vi "opCRD Server.vi"   [LabVIEW 2013]
uses:
  CRD/tCRD.lvclass
  Reusable/Instrument/state.ctl
  Reusable/Instrument/Instrument.lvclass
types:
  T1 = typedef "Instrument.lvclass/state.ctl" = enum8{"Configure", "Acquire", "Wait", "Quit", "Handle Error", "NOOP"}
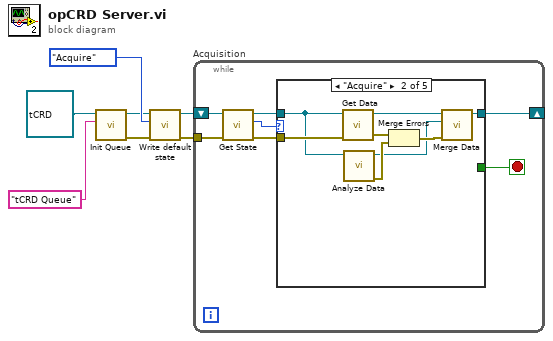
[diagram p0: block diagram]
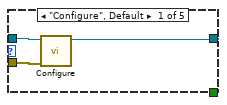
[diagram p2: hidden frame]
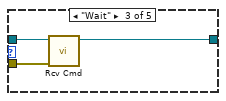
[diagram p3: hidden frame]
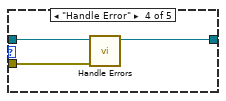
[diagram p4: hidden frame]
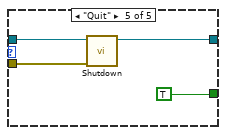
[diagram p5: hidden frame]
diagram:
  n1 = call "Init Queue.vi"("queue_name"="tCRD Queue", "Instrument in"=refnum<class "tCRD.lvclass"> refnum ("tCRD")) -> ("error out"=w1:errorcluster, "Instrument out"=w2:refnum<class "tCRD.lvclass">)  [unwired: 8 in]
  n2 = call "Write default state.vi"("error in (no error)"=w1, "instr state"=state."Acquire", "Instrument in"=w2) -> ("error out"=w3:errorcluster, "Instrument out"=w4:refnum<class "tCRD.lvclass">)  [unwired: 7 in]
  n3 = while "Acquisition" {
    tunnel: w3 -> [w14]
    shift-right: [w8] -> _
    shift-left: w4 -> [w12]
    stop <- w9 stop-if-true
    n4 = call "Get State.vi"("error in"=w14, "Instrument in"=w12) -> ("error out"=w10:errorcluster, "default state"=w13:T1, "Instrument out"=w11:refnum<class "tCRD.lvclass">)  [unwired: 7 in]
    n5 = case shown="\"Acquire\"" w13 {
      tunnel: w11 -> [w17 w18 w28 w31 w34]
      tunnel: w10 -> [w16 w25 w26 w30 w33]
      tunnel: [_ _ _ _ TRUE] -> w9
      tunnel: [w15 w21 w27 w29 w32] -> w8
      frame "Configure", Default {
        n6 = call-dynamic "Configure.vi"("error in"=w16, "tCRD in"=w17) -> ("tCRD out"=w15:refnum<class "tCRD.lvclass">)  [unwired: 8 in, 1 out]
      }
      frame "Acquire" {
        n7 = call-dynamic "Get Data.vi"("error in"=w25, "tCRD in"=w18) -> ("error out"=w24:errorcluster, "tCRD out"=w22:refnum<class "tCRD.lvclass">)  [unwired: 8 in]
        n8 = call-dynamic "Analyze Data.vi"("tCRD in"=w18) -> ("error out"=w23:errorcluster, "tCRD out"=w19:refnum<class "tCRD.lvclass">)  [unwired: 9 in]
        n9 = Merge Errors(w24, w23) -> (w20:errorcluster)
        n10 = call-dynamic "Merge Data.vi"("error in"=w20, "Analyzed"=w19, "Acquired"=w22) -> ("tCRD out"=w21:refnum<class "tCRD.lvclass">)  [unwired: 7 in, 1 out]
      }
      frame "Wait" {
        n11 = call-dynamic "Rcv Cmd.vi"("error in"=w26, "tCRD in"=w28) -> ("tCRD out"=w27:refnum<class "tCRD.lvclass">)  [unwired: 8 in, 1 out]
      }
      frame "Handle Error" {
        n12 = call-dynamic "Handle Errors.vi"("error in"=w30, "tCRD in"=w31) -> ("tCRD out"=w29:refnum<class "tCRD.lvclass">)  [unwired: 7 in, 2 out]
      }
      frame "Quit" {
        n13 = call-dynamic "Shutdown.vi"("error in"=w33, "tCRD in"=w34) -> ("tCRD out"=w32:refnum<class "tCRD.lvclass">)  [unwired: 8 in, 1 out]
      }
    }
  }
